vi "Run.vi"(8 "error in (no error)":errorcluster, 11 "Test Suite with Global Fixture In":refnum<class "Global Fixture Test Suite.lvclass">) -> (0 "error out":errorcluster, 1 "Done?":bool, 2 "Results":T1(array[cluster]), 3 "Test Suite with Global Fixture Out":refnum<class "Global Fixture Test Suite.lvclass">)   [LabVIEW 2020, in "Global Fixture Test Suite.lvclass"]
uses:
  Global Fixture Test Suite.lvclass
  Global Fixture Test Suite.lvclass/Global Fixture Test Suite.ctl
  Global Fixture Test Case/Global Fixture Test Case.lvclass
  <vilib>/Astemes/LUnit/Test Suite.lvclass
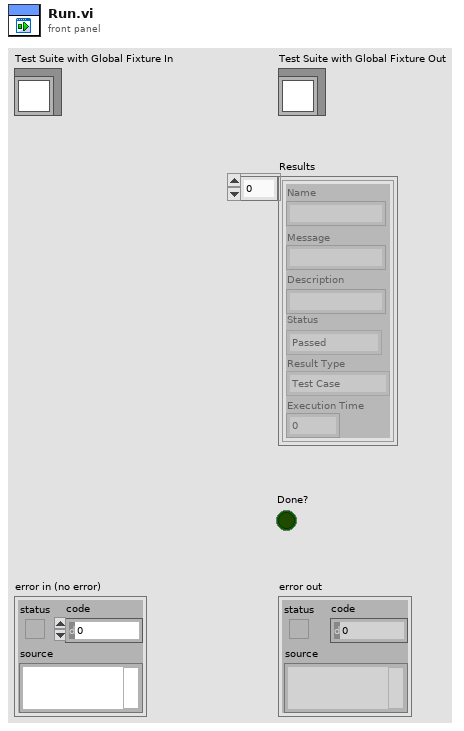
[diagram p1: front panel]
types:
  T1 = cluster{"Name":string, "Message":string, "Description":string, "Status":enum16{"", "Passed", "Failed", "Error", "Skipped", "Setup Error", "Broken", "Teardown Error"}, "Result Type":enum16{"Test Case", "Test Suite", "Test Run", "Pass", "Fail", "Skip", "Pass if", "Fail if", "Pass if Error", "Fail if Error", "Pass if Equal", "Fail if Equal"}, "Execution Time":dbl}[]
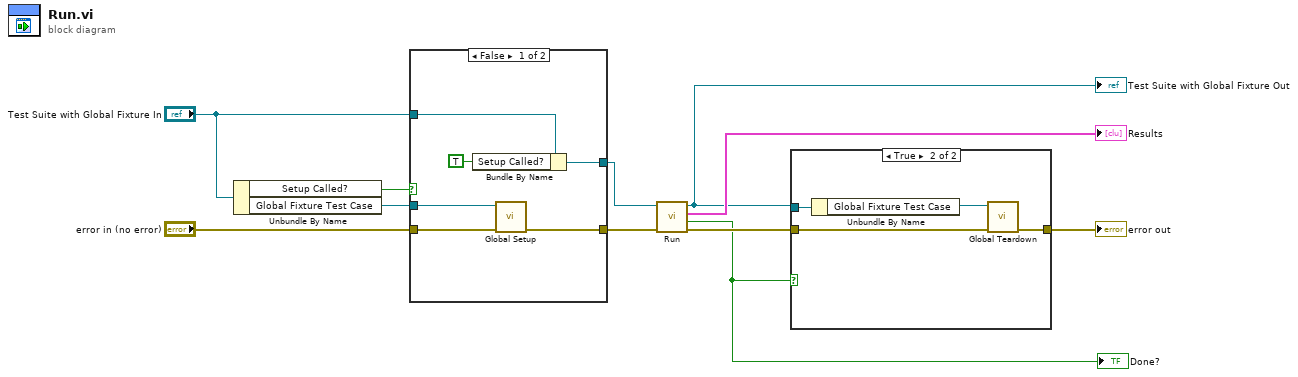
[diagram p0: block diagram]
diagram:
  n1 = Unbundle By Name("Test Suite with Global Fixture In") -> ("Setup Called?"=w1:bool, "Global Fixture Test Case"=w6:refnum<class "Global Fixture Test Case.lvclass">)
  n2 = case shown="False" w1 {
    tunnel: "error in (no error)" -> [w17 w18]
    tunnel: "Test Suite with Global Fixture In" -> [w16 w19]
    tunnel: [w15 w18] -> w7
    tunnel: w6 -> [w14 _]
    tunnel: [w13 w19] -> w3
    frame False {
      n3 = Bundle By Name(cluster=w16, "Setup Called?"=TRUE) -> (w13:refnum<class "Global Fixture Test Suite.lvclass">)
      n4 = call-dynamic "Global Setup.vi"("error in (no error)"=w17, "Global Fixture Test Case in"=w14) -> ("error out"=w15:errorcluster)  [unwired: 9 in]
    }
    frame True {
    }
  }
  n5 = call-parent "Run.vi"("error in (no error)"=w7, "LUnit Test Suite In"=w3) -> ("error out"=w11:errorcluster, "Done?"=w4:bool, "Results"=→"Results":T1, "LUnit Test Suite In 2"=w2:refnum<class "Global Fixture Test Suite.lvclass">)  [unwired: 6 in]
  "Test Suite with Global Fixture Out" <- w2
  "Done?" <- w4
  n6 = case shown="True" w4 {
    tunnel: w11 -> [w20 w24]
    tunnel: [w20 w23] -> w5
    tunnel: w2 -> [_ w21]
    frame False {
    }
    frame True {
      n7 = Unbundle By Name(w21) -> ("Global Fixture Test Case"=w22:refnum<class "Global Fixture Test Case.lvclass">)
      n8 = call-dynamic "Global Teardown.vi"("error in (no error)"=w24, "Global Fixture Test Case in"=w22) -> ("error out"=w23:errorcluster)  [unwired: 9 in]
    }
  }
  "error out" <- w5
